vi "Create Session.vi"(6 "timeout (ms)":i32=1000, 8 "error in (no error)":errorcluster) -> (0 "error out":errorcluster, 3 "session out":refnum<class "AudioGeneration.lvclass">)   [LabVIEW 2021, in "AudioGeneration.lvclass"]
uses:
  AudioGeneration.lvclass
  AudioGeneration.lvclass/AudioGeneration.ctl
  <vilib>/NI/STM/TCP/Read Meta Data (TCP Clst).vi
  <vilib>/NI/STM/TCP/Read Meta Data (TCP Ref).vi
  <vilib>/NI/STM/NI STM.lvlib
  subVIs/utility/AudioGenUtility.lvlib
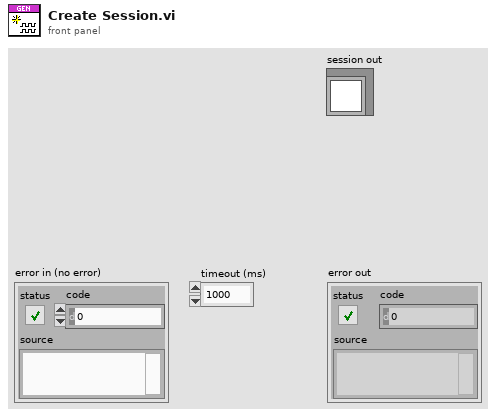
[diagram p1: front panel]
types:
  T1 = typedef "AudioGenTypeDefs.lvlib/service settings.ctl" = cluster{"port":u32, "enable debug log":bool}
  T2 = typedef "NI STM.lvlib/TCP Connection Info.ctl" = cluster{"connection ID":refnum<k5>, "meta data":T3[]}
  T3 = typedef "NI STM.lvlib/MetaDataElement.ctl" = string
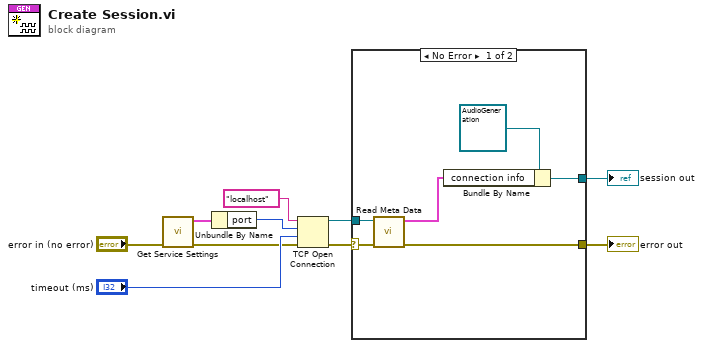
[diagram p0: block diagram]
diagram:
  n1 = call "Get Service Settings.vi"("error in (no error)"="error in (no error)") -> ("error out"=w3:errorcluster, "service settings"=w2:T1)  [unwired: 9 in]
  n2 = Unbundle By Name(w2) -> ("port"=w1:u32)
  n3 = TCP Open Connection(address="localhost" ("Target IP Address"), remote port or service name=w1, timeout ms (60000)="timeout (ms)", error in (no error)=w3) -> (connection ID=w7:refnum<k5>, error out=w8:errorcluster)  [unwired: 1 out]
  n4 = case shown="No Error" w8 {
    selector: w8 -> [w15 w17]
    tunnel: w7 -> [w14 _]
    tunnel: [w12 w17] -> w6
    tunnel: [w11 _] -> w5
    frame No Error {
      n5 = call-poly <vilib>:"Read Meta Data.vi"("error in"=w15, "connection ID"=w14) -> ("error out"=w12:errorcluster, "connection info out"=w13:T2)  [unwired: 1 in, 7 out]
      n6 = Bundle By Name(cluster=refnum<class "AudioGeneration.lvclass"> refnum ("session out"), "connection info"=w13) -> (w11:refnum<class "AudioGeneration.lvclass">)
    }
    frame Error {
    }
  }
  "error out" <- w6
  "session out" <- w5
